vi "FIB spot PXIe-6124.vi"(6 "Z center":dbl=-0.98 min=-1.0 max=1.0, 7 "X center":dbl=-0.98 min=-1.0 max=1.0, 8 "FIB Scan Parameters":T1={"X resolution"=512, "Z resolution"=512, "X center"=0.0, "Z center"=0.0, "X size (V)"=20.0, "Z size (V)"=20.0, "Frame line rampdown ratio"=-0.1, "Scan rate (Hz)"=2000000, "Oversampling"=2} {"Z size (V)" min=0.0 max=20.0; "X size (V)" min=0.0 max=20.0; "Frame line rampdown ratio" min=-1.0 max=1.0 step=0.05 format="%.2g"; "Scan rate (Hz)" max=4000000 format="%#.6p"; "Z resolution" max=2048; "X resolution" max=2048}, 10 "Options":cluster{"Flip x":bool, "Flip z":bool}={"Flip x"=TRUE, "Flip z"=TRUE}, 11 "HW Config":T2={"FIB X coil"="PXI1Slot7/ao0", "FIB Y coil"="PXI1Slot7/ao1", "Beam blank"="PXI1Slot7/port0/line0", "Ext scan"="PXI1Slot7/port0/line0", "Detector"="PXI1Slot7/ai0", "Post #1up"="PXI1Slot2/ao0", "Post #1down"="PXI1Slot2/ao1", "Post #2up"="PXI1Slot2/ao2", "Post #2down"="PXI1Slot2/ao3"}) -> (0 "error out":errorcluster)   [LabVIEW 2018]
uses:
  <vilib>/DAQmx/write.llb/DAQmx Write (Analog 2D DBL NChan NSamp).vi
  <vilib>/DAQmx/create/channels.llb/DAQmx Create Channel (AO-Voltage-Basic).vi
  <vilib>/DAQmx/configure/timing.llb/DAQmx Timing (Sample Clock).vi
  <vilib>/DAQmx/miscellaneous.llb/DAQmx Fill In Error Info.vi
  <resource>/objmgr/daqmx.rc
panel:
  in  "Api":refnum<k7>(container)
  out "Low blanked":bool
  in  "Machine Type":u8(ring) items=["Feiss", "NVision", "Jeiss"]
  out "Ext scan":tag
  out "FIB Y coil":tag
  out "FIB X coil":tag
  out "Beam blank":tag
  in  "spot":bool
  # "Scan coils"
  # "Flip"
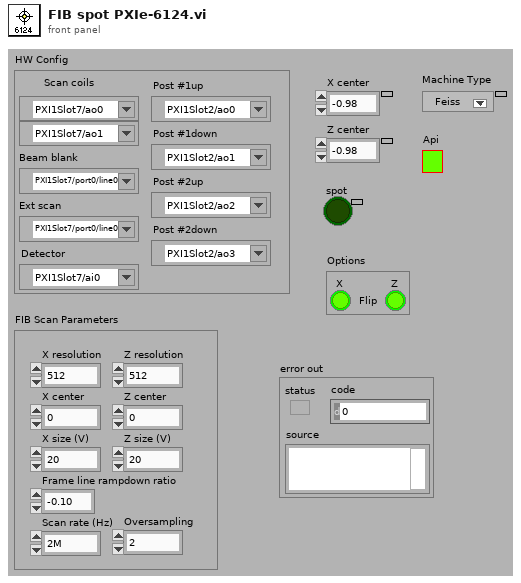
[diagram p1: front panel]
types:
  T1 = cluster{"X resolution":u32, "Z resolution":u32, "X center":dbl, "Z center":dbl, "X size (V)":dbl, "Z size (V)":dbl, "Frame line rampdown ratio":dbl, "Scan rate (Hz)":u32, "Oversampling":u16}
  T2 = cluster{"FIB X coil":tag, "FIB Y coil":tag, "Beam blank":tag, "Ext scan":tag, "Detector":tag, "Post #1up":tag, "Post #1down":tag, "Post #2up":tag, "Post #2down":tag}
  T3 = enum16{"SEM", "FIB", "Mill", "SEM + FIB", "Mill + SEM", "Drift SEM", "Drift FIB", "None", "Ext", "Ext + SEM"}
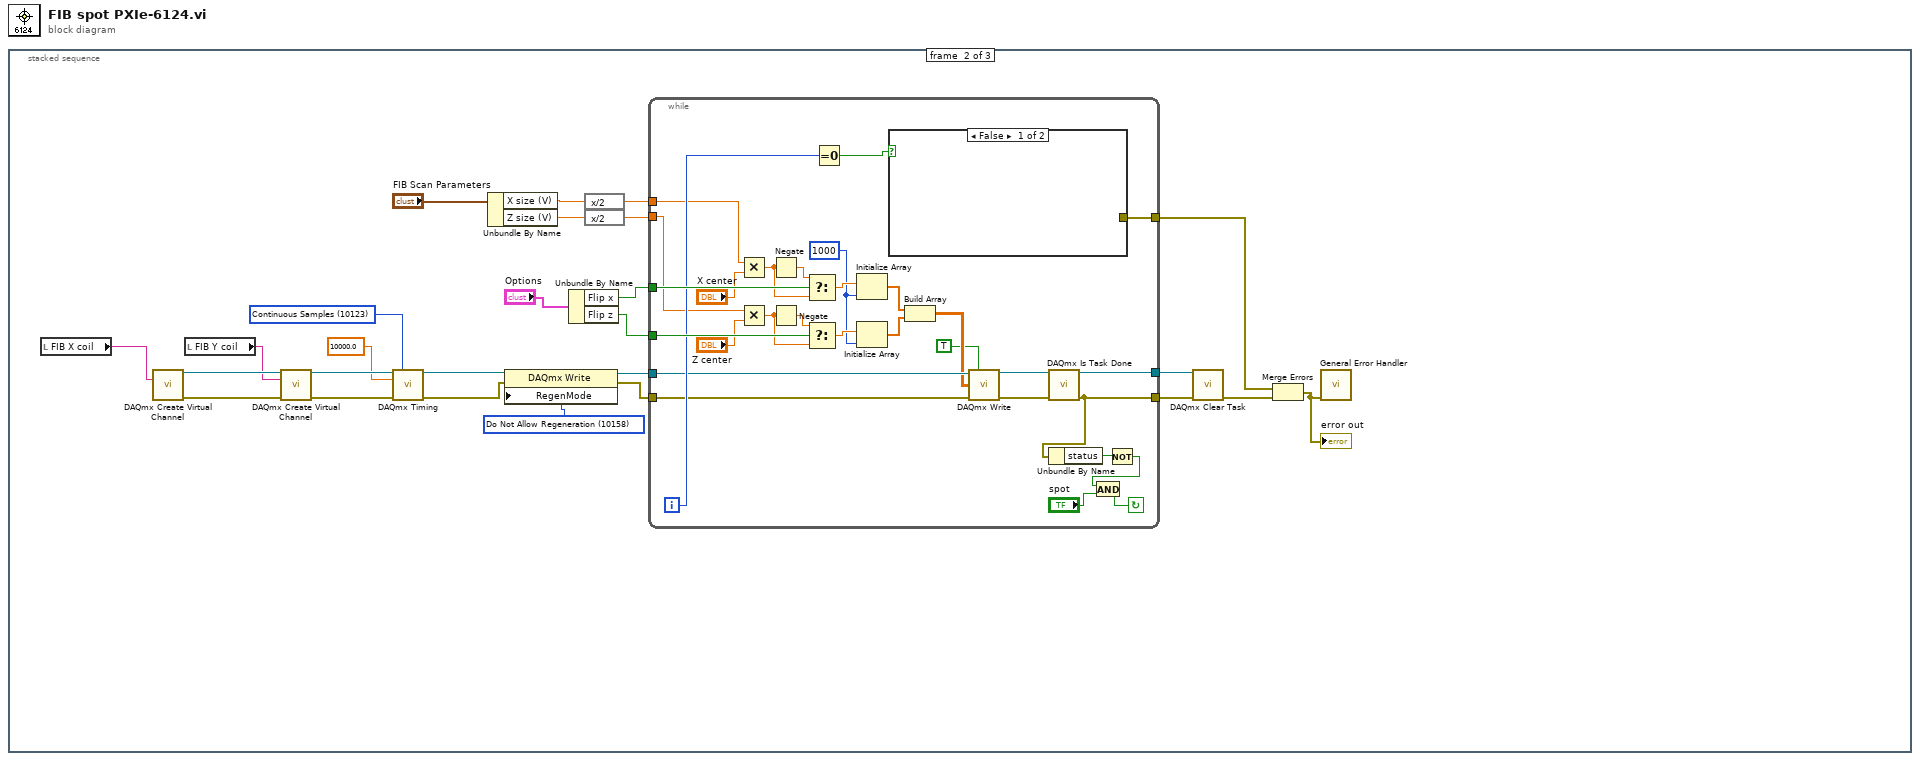
[diagram p0: block diagram]
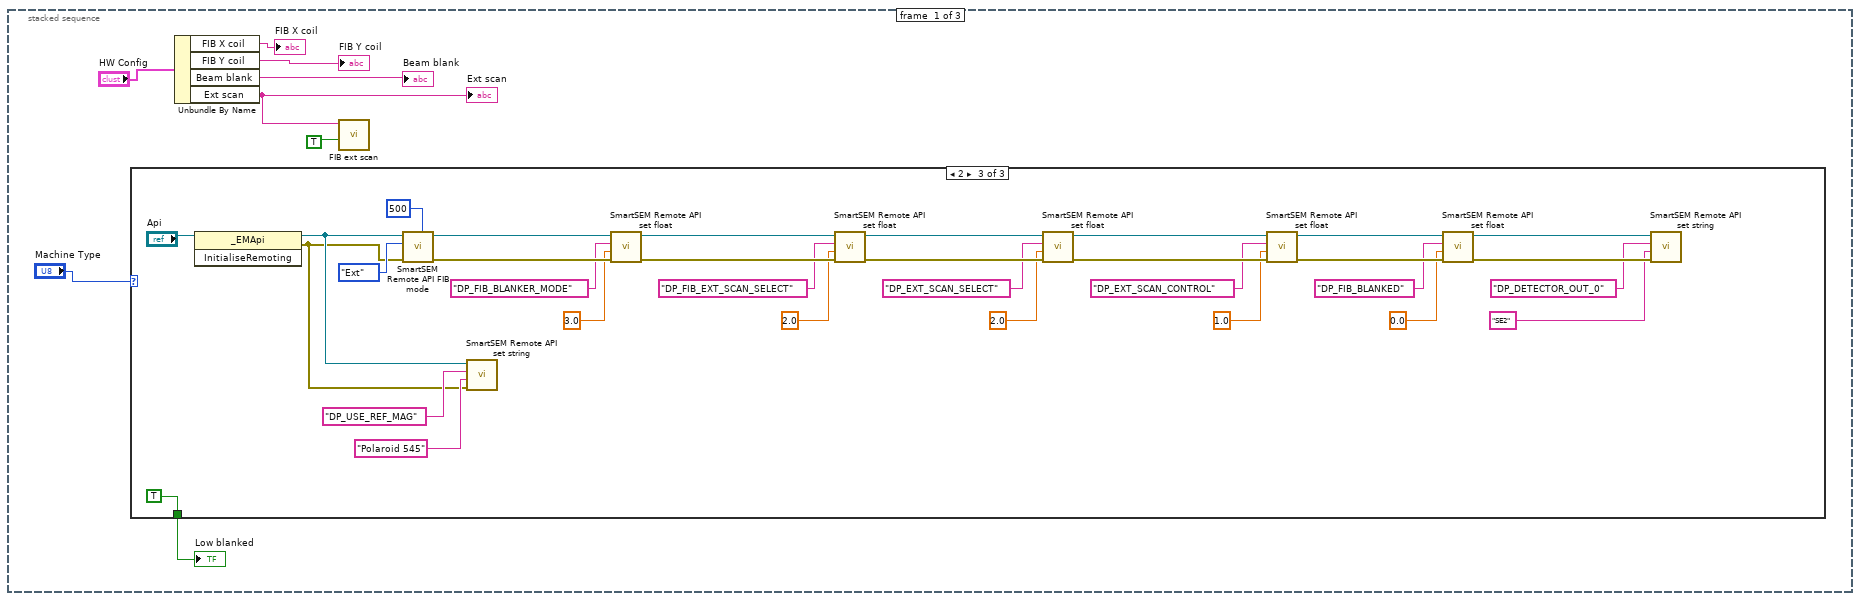
[diagram p2: hidden frame]
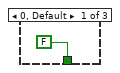
[diagram p3: hidden frame]
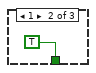
[diagram p4: hidden frame]
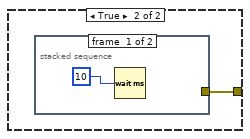
[diagram p5: hidden frame]
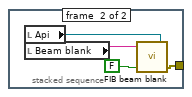
[diagram p6: hidden frame]
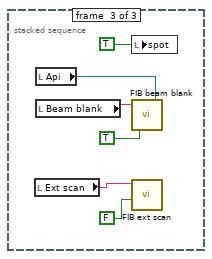
[diagram p7: hidden frame]
diagram:
  n1 = stacked-sequence {
    frame #0 {
      n2 = case shown="2" "Machine Type" {
        tunnel: [FALSE ("Beam blanked") TRUE ("Beam blanked") TRUE ("Beam blanked")] -> w1
        frame 0, Default {
        }
        frame 1 {
        }
        frame 2 {
          n3 = invoke class="_EMApi" method="InitialiseRemoting"(reference="Api") -> (reference out=w13:refnum<k7>, error out=w12:errorcluster)  [unwired: 2 in, 1 out]
          n4 = call "SmartSEM Remote API FIB mode.vi"("Wait (ms)"=u32 500, "error in"=w12, "FIB mode"=T3."Ext", "Api"=w13) -> ("error out"=w36:errorcluster, "Api out"=w37:refnum<k7>)  [unwired: 6 in]
          n5 = call "SmartSEM Remote API set string.vi"("error in"=w12, "vValue"="Polaroid 545" ("lpszParam"), "lpszParam"="DP_USE_REF_MAG", "Api"=w13) -> ()  [unwired: 6 in, 2 out]
          n6 = call "SmartSEM Remote API set float.vi"("error in"=w36, "vValue"=sgl 3.0, "lpszParam"="DP_FIB_BLANKER_MODE", "Api"=w37) -> ("error out"=w32:errorcluster, "Api out"=w33:refnum<k7>)  [unwired: 6 in]
          n7 = call "SmartSEM Remote API set float.vi"("error in"=w32, "vValue"=sgl 2.0, "lpszParam"="DP_FIB_EXT_SCAN_SELECT" ("lpszCommand"), "Api"=w33) -> ("error out"=w28:errorcluster, "Api out"=w29:refnum<k7>)  [unwired: 6 in]
          n8 = call "SmartSEM Remote API set float.vi"("vValue"=sgl 2.0, "lpszParam"="DP_EXT_SCAN_SELECT" ("lpszCommand")) -> ()  [unwired: 8 in, 2 out]
          n9 = call "SmartSEM Remote API set float.vi"("error in"=w28, "vValue"=sgl 1.0, "lpszParam"="DP_EXT_SCAN_CONTROL" ("lpszCommand"), "Api"=w29) -> ("error out"=w24:errorcluster, "Api out"=w25:refnum<k7>)  [unwired: 6 in]
          n10 = call "SmartSEM Remote API set float.vi"("error in"=w24, "vValue"=sgl 0.0, "lpszParam"="DP_FIB_BLANKED", "Api"=w25) -> ("error out"=w20:errorcluster, "Api out"=w21:refnum<k7>)  [unwired: 6 in]
          n11 = call "SmartSEM Remote API set string.vi"("error in"=w20, "vValue"="SE2" ("Det A Type"), "lpszParam"="DP_DETECTOR_OUT_0", "Api"=w21) -> ()  [unwired: 6 in, 2 out]
        }
      }
      "Low blanked" <- w1
      n12 = Unbundle By Name("HW Config") -> ("FIB X coil"=→"FIB X coil":tag, "FIB Y coil"=→"FIB Y coil":tag, "Beam blank"=→"Beam blank":tag, "Ext scan"=w3:tag)
      "Ext scan" <- w3
      n13 = call "FIB ext scan.vi"("Ext on"=TRUE ("data"), "FIB Ext Scan"=w3) -> ()  [unwired: 9 in, 1 out]
    }
    frame #1 {
      w53 = 10123 items=["Finite Samples"=10178, "Continuous Samples"=10123, "Hardware Timed Single Point"=12522] ("sample mode")
      w60 = 10158 items=["Allow Regeneration"=10097, "Do Not Allow Regeneration"=10158] ("RegenMode")
      n14 = local read "FIB X coil"() -> (w55:tag)
      n15 = call-poly <vilib>:"DAQmx Create Virtual Channel.vi"("physical channels"=w55) -> ("task out"=w58:refnum<k21>, "error out"=w59:errorcluster)  [unwired: 8 in, 5 out]
      n16 = local read "FIB Y coil"() -> (w54:tag)
      n17 = call-poly <vilib>:"DAQmx Create Virtual Channel.vi"("task in"=w58, "physical channels"=w54, "error in"=w59) -> ("task out"=w56:refnum<k21>, "error out"=w57:errorcluster)  [unwired: 6 in, 5 out]
      n18 = call-poly <vilib>:"DAQmx Timing.vi"("task/channels in"=w56, "sample mode"=w53, "rate"=10000.0, "error in"=w57) -> ("task out"=w61:refnum<k21>, "error out"=w62:errorcluster)  [unwired: 3 in, 7 out]
      n19 = Unbundle By Name("FIB Scan Parameters") -> ("X size (V)"=w44:dbl, "Z size (V)"=w43:dbl)
      n20 = property class="DAQmx Write"(reference=w61, error in=w62, "RegenMode"=w60) -> (reference out=w50:refnum<k21>, error out=w49:errorcluster)
      n21 = Unbundle By Name("Options") -> ("Flip x"=w63:bool, "Flip z"=w64:bool)
      n22 = expression code="x/2"(w44) -> (w42:dbl)
      n23 = expression code="x/2"(w43) -> (w41:dbl)
      n24 = while {
        tunnel: [w92] -> w65
        tunnel: w64 -> [w89]
        tunnel: w63 -> [w88]
        tunnel: w50 -> [w83]
        tunnel: w49 -> [w82]
        tunnel: [w81] -> w48
        tunnel: [w80] -> w47
        tunnel: w42 -> [w70]
        tunnel: w41 -> [w68]
        i -> [w87]
        stop <- w95 continue-if-true
        w77 = 1000 ("dimension size")
        n25 = Multiply(x=w70, y="X center") -> (x*y=w71:dbl)
        n26 = Multiply(x=w68, y="Z center") -> (x*y=w67:dbl)
        n27 = Negate(x=w71) -> (-x=w91:dbl)
        n28 = Negate(x=w67) -> (-x=w90:dbl)
        n29 = Select(t=w91, s=w88, f=w71) -> (s? t:f=w79:dbl)
        n30 = Select(t=w90, s=w89, f=w67) -> (s? t:f=w78:dbl)
        n31 = Equal To 0?(x=w87) -> (x = 0?=w86:bool)
        n32 = Initialize Array(w79, w77) -> (w76:dbl[])
        n33 = Initialize Array(w78, w77) -> (w75:dbl[])
        n34 = case shown="False" w86 {
          tunnel: [_ w97] -> w92
          frame False {
          }
          frame True {
            n35 = stacked-sequence {
              tunnel: [_ w100] -> w97
              frame #0 {
                n36 = Wait (ms)(milliseconds to wait=u32 10) -> ()  [unwired: 1 out]
              }
              frame #1 {
                n37 = local read "Api"() -> (w99:refnum<k7>)
                n38 = local read "Beam blank"() -> (w102:tag)
                n39 = call "FIB beam blank.vi"("Api"=w99, "Beam blanked"=FALSE, "lines"=w102) -> ("error out"=w100:errorcluster)  [unwired: 2 in]
              }
            }
          }
        }
        n40 = Build Array(w76, w75) -> (w74:dbl[][])
        n41 = call-poly <vilib>:"DAQmx Write.vi"("task/channels in"=w83, "auto start"=TRUE, "data"=w74, "error in"=w82) -> ("task out"=w84:refnum<k21>, "error out"=w85:errorcluster)  [unwired: 10 out]
        n42 = call <vilib>:"DAQmx Is Task Done.vi"("task/channels in"=w84, "error in"=w85) -> ("task out"=w81:refnum<k21>, "error out"=w80:errorcluster)  [unwired: 2 in, 10 out]
        n43 = Unbundle By Name(w80) -> ("status"=w94:bool)
        n44 = Not(x=w94) -> (.not. x?=w93:bool)
        n45 = And(x=w93, y="spot") -> (x .and. y?=w95:bool)
      }
      n46 = call <vilib>:"DAQmx Clear Task.vi"("task in"=w48, "error in"=w47) -> ("error out"=w46:errorcluster)  [unwired: 13 out]
      n47 = Merge Errors(w65, w46) -> (w66:errorcluster)
      "error out" <- w66
      n48 = call <vilib>:"General Error Handler.vi"("error in (no error)"=w66) -> ()  [unwired: 10 in, 5 out]
    }
    frame #2 {
      n49 = local read "Ext scan"() -> (w105:tag)
      n50 = local read "Api"() -> (w103:refnum<k7>)
      n51 = local read "Beam blank"() -> (w107:tag)
      n52 = local write "spot"(TRUE ("stop")) -> ()
      n53 = call "FIB beam blank.vi"("Api"=w103, "Beam blanked"=TRUE, "lines"=w107) -> ()  [unwired: 2 in, 1 out]
      n54 = call "FIB ext scan.vi"("Ext on"=FALSE ("data"), "FIB Ext Scan"=w105) -> ()  [unwired: 9 in, 1 out]
    }
  }
